vi "Set pins on switch board.vi"(8 "Error In":errorcluster, 11 "Experiment type":u16(ring) items=["PCB-Keithley", "PCB-EQE", "Manual-Keithley", "Manual-EQE"]) -> (0 "error out":errorcluster)   [LabVIEW 2011]
uses:
  <vilib>/MakerHub/LINX/Public/Peripherals/Digital/Digital Write N Chans.vi
  <vilib>/MakerHub/LINX/LMH-LINX.lvlib
panel:
  in  "Manual Enable Channel":u8=4
  out "Serial Port out":refnum<visa-resource-name>="COM3"
  in  "PCB Enable Channel":u8=5
  in  "A0 Channel":u8=6
  in  "A1 Channel":u8=7
  in  "Serial Port":refnum<visa-resource-name>="COM6"
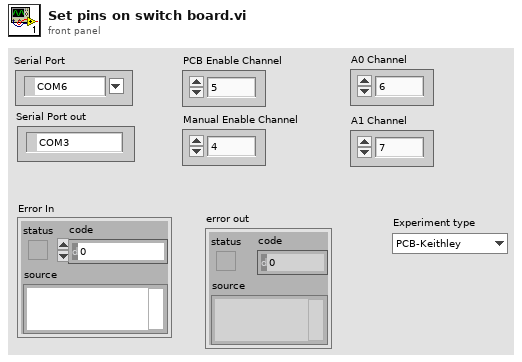
[diagram p1: front panel]
types:
  T1 = typedef "LMH-LINX.lvlib/LINX Ref.ctl" = cluster{"Platform":T2, "Interface":T3, "LINX Device Config":T4}
  T2 = typedef "LMH-LINX.lvlib/Platform.ctl" = enum16{"LINX", "myRIO"}
  T3 = typedef "LMH-LINX.lvlib/Interface.ctl" = enum16{"Serial", "TCP"}
  T4 = typedef "LMH-LINX.lvlib/Device.lvlib/LINX Device Config.ctl" = cluster{"Interface":T3, "COM Port":refnum<visa-resource-name>, "TCP Configuration":T5, "Device Family":u8, "Device ID":u8, "Device Name":string, "TCP Ref":refnum<k5>, "Channels":T6}
  T5 = typedef "LMH-LINX.lvlib/Device.lvlib/TCP Config.ctl" = cluster{"IP Address":string, "Port":u16}
  T6 = typedef "LMH-LINX.lvlib/Channels.ctl" = cluster{"DI":u8[], "DO":u8[], "AI":u8[], "AO":u8[], "PWM":u8[], "QE":u8[], "UART":u8[], "I2C 2":u8[], "SPI":u8[], "CAN":u8[], "Servo":u8[], "AI Ref (V)":dbl, "AO Ref (V)":dbl, "AO Resolution (Bits)":u8}
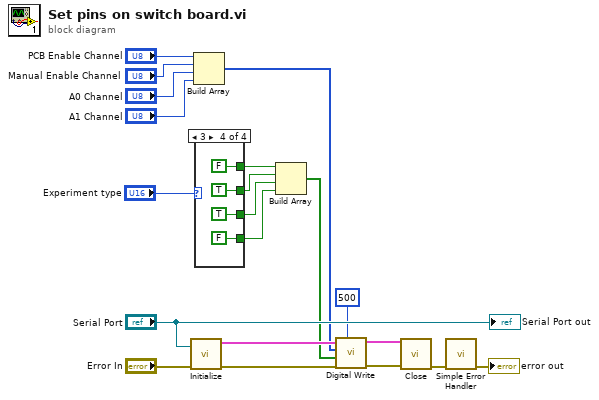
[diagram p0: block diagram]
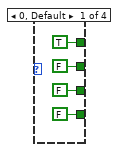
[diagram p2: hidden frame]
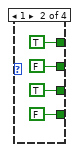
[diagram p3: hidden frame]
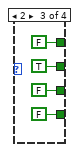
[diagram p4: hidden frame]
diagram:
  n1 = call <vilib>:"Initialize.vi"("Serial Port"="Serial Port", "Error In"="Error In") -> ("Error Out"=w13:errorcluster, "LINX Ref"=w14:T1)  [unwired: 7 in, 1 out]
  n2 = Build Array("PCB Enable Channel", "Manual Enable Channel", "A0 Channel", "A1 Channel") -> (w10:u8[])
  n3 = case shown="3" "Experiment type" {
    tunnel: [TRUE TRUE FALSE FALSE] -> w6
    tunnel: [FALSE FALSE TRUE TRUE] -> w5
    tunnel: [FALSE TRUE FALSE TRUE] -> w4
    tunnel: [FALSE FALSE FALSE FALSE] -> w3
    frame 0, Default {
    }
    frame 1 {
    }
    frame 2 {
    }
    frame 3 {
    }
  }
  n4 = Build Array(w6, w5, w4, w3) -> (w2:bool[])
  n5 = call-poly <vilib>:"Digital Write.vi"("Timeout (100 ms)"=500, "Error In"=w13, "Values"=w2, "DO Channels"=w10, "LINX Resource"=w14) -> ("Error Out"=w18:errorcluster, "LINX Resource"=w19:T1)  [unwired: 5 in]
  n6 = call <vilib>:"Close.vi"("Error In"=w18, "LINX Resource"=w19) -> ("Error Out"=w20:errorcluster)  [unwired: 8 in, 1 out]
  n7 = call <vilib>:"Simple Error Handler.vi"("error in (no error)"=w20) -> ("error out"=→"error out":errorcluster)  [unwired: 4 in, 4 out]
  "Serial Port out" <- "Serial Port"
